vi "Show Cursors.vi"(6 "Cursor Options":T1={"font"={"Font Name"="Arial", "Size"=14, "Strikeout?"=FALSE, "Italic?"=FALSE, "Underline?"=FALSE, "Outline?"=FALSE, "Shadow?"=FALSE, "Bold?"=FALSE}, "size"=1, "Timestamp"=enum."at TOP", "Vertical Line?"=FALSE, "Horizontal Line?"=FALSE, "alignment(left, top)"={"horizontal"=enum."center", "vertical"=enum."center"}, "TextFormat"="%2$.2f\\n\\n%1$s", "time format (%H:%M:%S)"="%H:%M%:S"} {"size" min=1 max=50}, 8 "error in (no error)":errorcluster, 9 "Coords":T2, 10 "XY Graph":refnum<vi>, 11 "input picture":picture) -> (0 "error out":errorcluster, 3 "output picture":picture)   [LabVIEW 2020, in "Graph Extensions.lvlib"]
doc: "Shows real time cursors overlayed in a graph, using just one mouse move event case. The options for the cursors can be highly customized to set up a unique cursor style.\n\nUsage: Place this inside an event structure on any XY graph, in the \"Mouse Move\" event case. Set the options as an input cluster to override the defaults. The output picture control would typically be connected to the XY Graph's \"PlotImages.Front\" property item.\n\nCursor Options\n<b>Horizontal Line?</b> - Draws a horizontal line to intersect each plot\n<b>Verticle Line?</b> - Draws a verticle line at the mouse location to highlight the cursor location (typically on the time scale)\n<b>Timestamp</b> - Sets where to display the timestamp (if you want it at the top or bottom) Used best with the verticle line turned on.\n<b>Font</b> - Setup the font for displaying the cursor text\n<b>Alignment</b> - Sets the alignment options for the text relative to the cursor point\n<b>TextFormat</b> - Sets the text display format at the cursor points to show. Three input parameters are available for the text, which can be accessed using parameter numbers.\ninputs: \n1$ - Timestamp at cursor locations\n2$ - Value of the plot\n3$ - Name of the plot\n\nExamples: $2$.2f\\n\\n%1$s\nThis shows the value of the plot with 2 decimal places. A blank line, then the name of the plot"
uses:
  Graph Extensions.lvlib
  <vilib>/Utility/miscctls.llb/LVPoint32TypeDef.ctl
  controls/CursorOptions.ctl
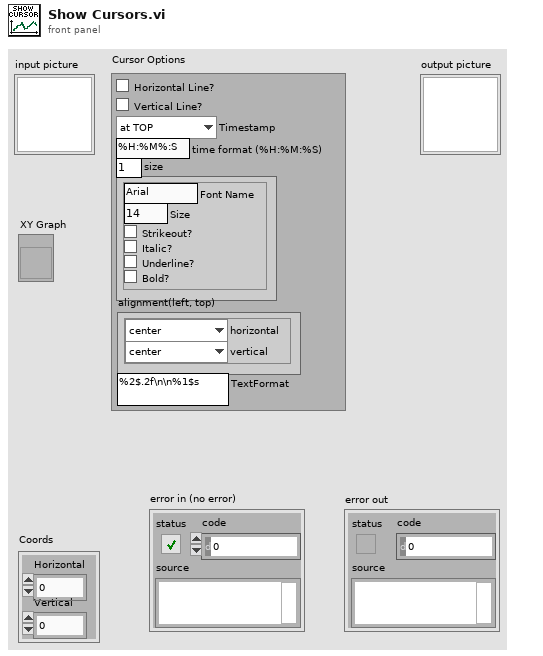
[diagram p1: front panel]
types:
  T1 = typedef "Graph Extensions.lvlib/CursorOptions.ctl" = cluster{"font":cluster{"Font Name":string, "Size":i16, "Strikeout?":bool, "Italic?":bool, "Underline?":bool, "Outline?":bool, "Shadow?":bool, "Bold?":bool}, "size":i16, "Timestamp":enum16{"at TOP", "at BOTTOM", "none"}, "Vertical Line?":bool, "Horizontal Line?":bool, "alignment(left, top)":cluster{"horizontal":enum16{"left", "center", "right"}, "vertical":enum16{"top", "center", "bottom"}}, "TextFormat":string, "time format (%H:%M:%S)":string}
  T2 = typedef "LVPoint32TypeDef.ctl" = cluster{"Horizontal":i32, "Vertical":i32}
  T3 = enum16{"User-specified Font", "Application Font", "System Font", "Dialog Font"}
  T4 = cluster{"horizontal":enum16{"left", "center", "right"}, "vertical":enum16{"top", "center", "bottom"}}
  T5 = cluster{"Font Name":string, "Size":i16, "Strikeout?":bool, "Italic?":bool, "Underline?":bool, "Outline?":bool, "Shadow?":bool, "Bold?":bool}
  T6 = typedef "LVRectTypeDef.ctl" = cluster{"Left":i16, "Top":i16, "Right":i16, "Bottom":i16}
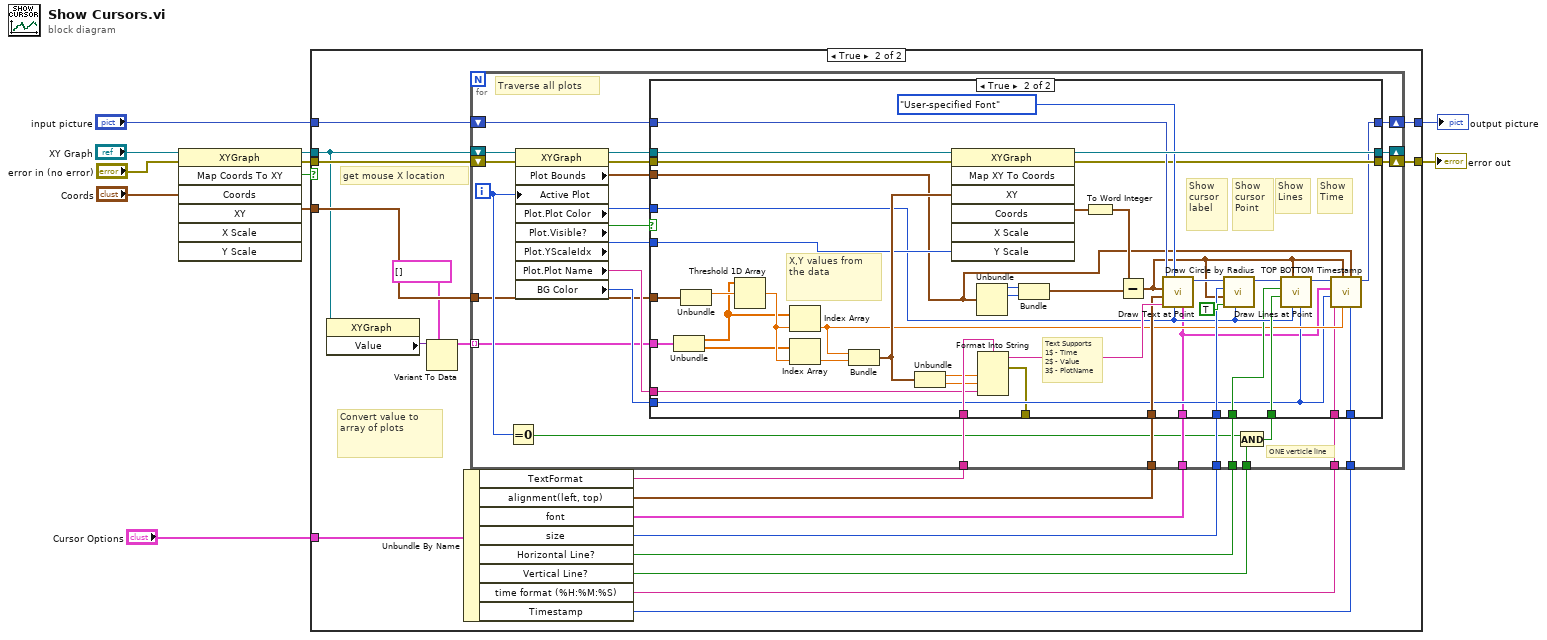
[diagram p0: block diagram]
diagram:
  n1 = invoke on="Invoke Node" class="XYGraph" method="Map Coords To XY"(reference="XY Graph", error in="error in (no error)", "Coords"="Coords") -> (reference out=w8:refnum<vi>, error out=w7:errorcluster, "Map Coords To XY"=w10:bool, "XY"=w11:cluster{"X":dbl, "Y":dbl})  [unwired: 4 in, 3 out]
  n2 = case shown="True" w10 {
    tunnel: w11 -> [_ w31]
    tunnel: w8 -> [_ w14]
    tunnel: [w12 w30] -> w3
    tunnel: w7 -> [w13 w29]
    tunnel: [w13 w28] -> w6
    tunnel: "input picture" -> [w12 w27]
    tunnel: "Cursor Options" -> [_ w19]
    frame False {
      # "not in plot area.  clear the image"
    }
    frame True {
      # "Convert value to array of plots"
      # "get mouse X location"
      n3 = property class="XYGraph"(reference=w14) -> ("Value"=w16:variant)  [unwired: 1 in, 2 out]
      n4 = Variant To Data(type=cluster{dbl[], dbl[]}[] [], Variant=w16) -> (data=w18:cluster{dbl[], dbl[]}[])  [unwired: 1 in, 1 out]
      n5 = Unbundle By Name(w19) -> ("TextFormat"=w26:string, "alignment(left, top)"=w25:T4, "font"=w24:T5, "size"=w23:i16, "Horizontal Line?"=w22:bool, "Vertical Line?"=w21:bool, "time format (%H:%M:%S)"=w15:string, "Timestamp"=w20:enum16{"at TOP", "at BOTTOM", "none"})
      n6 = for {
        tunnel: w18 -> [w33] mode=indexing
        shift-right: [w57] -> _
        shift-left: w14 -> [w55]
        tunnel: w31 -> [w34]
        shift-right: [w53] -> w30
        shift-left: w27 -> [w56]
        shift-right: [w48] -> w28
        shift-left: w29 -> [w50]
        tunnel: w23 -> [w46]
        tunnel: w25 -> [w45]
        tunnel: w24 -> [w44]
        tunnel: w26 -> [w43]
        tunnel: w22 -> [w42]
        tunnel: w21 -> [w38]
        tunnel: w20 -> [w36]
        tunnel: w15 -> [w32]
        i -> [w41]
        # "Traverse all plots"
        # "ONE verticle line"
        n7 = Equal To 0?(x=w41) -> (x = 0?=w39:bool)
        n8 = property on="Property Node" class="XYGraph"(reference=w55, error in=w50, "Active Plot"=w41) -> (reference out=w54:refnum<vi>, error out=w49:errorcluster, "Plot Bounds"=w58:T6, "Plot.Plot Color"=w52:u32, "Plot.Visible?"=w51:bool, "Plot.YScaleIdx"=w47:u32, "Plot.Plot Name"=w37:string, "BG Color"=w35:u32)
        n9 = And(x=w39, y=w38) -> (x .and. y?=w40:bool)
        n10 = case shown="True" w51 {
          tunnel: w58 -> [_ w67]
          tunnel: [w61 w99] -> w57
          tunnel: w33 -> [_ w94]
          tunnel: w34 -> [_ w93]
          tunnel: w56 -> [w60 w92]
          tunnel: w54 -> [w61 w89]
          tunnel: [w60 w72] -> w53
          tunnel: w52 -> [_ w77]
          tunnel: w49 -> [w59 w85]
          tunnel: [w59 w84] -> w48
          tunnel: w47 -> [_ w83]
          tunnel: w46 -> [_ w82]
          tunnel: w45 -> [_ w81]
          tunnel: w44 -> [_ w65]
          tunnel: w43 -> [_ w80]
          tunnel: w42 -> [_ w76]
          tunnel: w40 -> [_ w79]
          tunnel: w37 -> [_ w73]
          tunnel: w36 -> [_ w69]
          tunnel: w35 -> [_ w66]
          tunnel: [_ w63] -> _
          tunnel: w32 -> [_ w62]
          frame False {
            # "plot is not visible, so don't show the cursor for it."
          }
          frame True {
            # "Show\nTime"
            # "Show\nLines"
            # "Show\ncursor\nPoint"
            # "Show\ncursor\nlabel"
            # "Text Supports\n1$ - Time\n2$ - Value\n3$ - PlotName"
            # "X,Y values from the data"
            n11 = Unbundle(w94) -> (w64:dbl[], w96:dbl[])
            n12 = Unbundle(w93) -> ("X"=w95:dbl)  [unwired: 1 out]
            n13 = Threshold 1D Array(2:w95, 3:w64) -> (0:w97:dbl)  [unwired: 1 in]
            n14 = Index Array(array=w64, index=w97) -> (element=w70:dbl)
            n15 = Index Array(array=w96, index=w97) -> (element=w98:dbl)
            n16 = Bundle("X"=w70, "X"=w98) -> (w91:cluster{"X":dbl, "X":dbl})  [unwired: 1 in]
            n17 = Unbundle(w91) -> ("X"=w75:dbl, "X"=w74:dbl)
            n18 = invoke on="Invoke Node" class="XYGraph" method="Map XY To Coords"(reference=w89, error in=w85, "XY"=w91, "Y Scale"=w83) -> (reference out=w99:refnum<vi>, error out=w84:errorcluster, "Coords"=w104:T2)  [unwired: 3 in, 4 out]
            n19 = Unbundle(w67) -> ("Left"=w102:i16, "Top"=w103:i16)  [unwired: 2 out]
            n20 = Format Into String(format string=w80, w75, w74, w73) -> (resulting string=w90:string, error out=w63:errorcluster)  [unwired: 2 in]
            n21 = Bundle("Left"=w102, "Top"=w103) -> (w100:cluster{"Left":i16, "Top":i16})  [unwired: 1 in]
            n22 = To Word Integer(number=w104) -> (16bit integer=w101:cluster{"Horizontal":i16, "Vertical":i16})
            n23 = Subtract(x=w101, y=w100) -> (x-y=w68:cluster{i16, i16})
            n24 = call <vilib>:"Draw Text at Point.vi"("[user-specified font]"=w65, "text color(black)"=w77, "desired font(Application)"=T3."User-specified Font", "text"=w90, "alignment(left, top)"=w81, "origin"=w68, "picture"=w92) -> ("new picture"=w88:picture)  [unwired: 3 in, 1 out]
            n25 = call <vilib>:"Draw Circle by Radius.vi"("color(black)"=w77, "fill?(F)"=TRUE, "pixel center"=w68, "radius"=w82, "picture"=w88) -> ("new picture"=w78:picture)  [unwired: 6 in]
            n26 = call "Draw Lines at Point.vi"("GraphBGK"=w66, "color(black)"=w77, "pixel center"=w68, "Vertical Line?"=w79, "Horizontal Line?"=w76, "new picture in"=w78) -> ("new picture out"=w71:picture)  [unwired: 5 in]
            n27 = call "TOP BOTTOM Timestamp.vi"("Format"=w69, "Rect"=w67, "Timestamp"=w70, "pixel center"=w68, "time format (%H:%M:%S)"=w62, "GraphBGK"=w66, "font"=w65, "new picture in"=w71) -> ("new picture out"=w72:picture)  [unwired: 3 in]
          }
        }
      }
    }
  }
  "error out" <- w6
  "output picture" <- w3
